vi "y轴排序.vi"(3 "均值角点":cluster{"X":sgl, "Y":sgl}[](array[cluster])) -> (1 "数组 2":cluster{"X":sgl, "Y":sgl}[](array[cluster]))   [LabVIEW 2018]
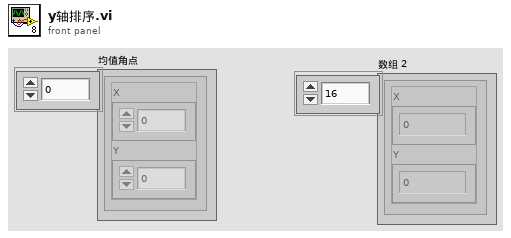
[diagram p1: front panel]
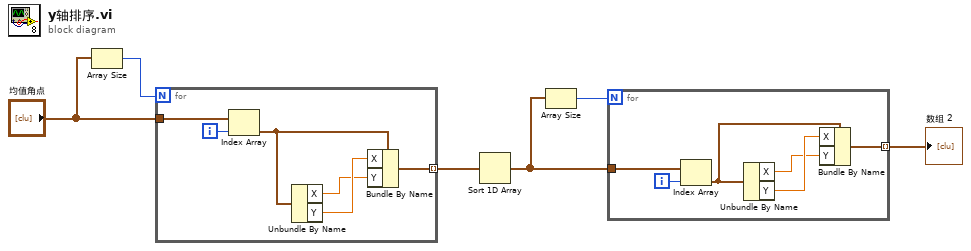
[diagram p0: block diagram]
diagram:
  n1 = Array Size(array="均值角点") -> (size(s)=w5:i32)
  n2 = for {
    N: w5 -> [_]
    tunnel: [w8] -> w4 mode=indexing
    tunnel: "均值角点" -> [w7]
    i -> [w12]
    n3 = Index Array(array=w7, index=w12) -> (element=w9:cluster{"X":sgl, "Y":sgl})
    n4 = Unbundle By Name(w9) -> ("X"=w10:sgl, "Y"=w11:sgl)
    n5 = Bundle By Name(cluster=w9, "X"=w11, "Y"=w10) -> (w8:cluster{"X":sgl, "Y":sgl})
  }
  n6 = Sort 1D Array(array=w4) -> (sorted array=w2:cluster{"X":sgl, "Y":sgl}[])
  n7 = Array Size(array=w2) -> (size(s)=w3:i32)
  n8 = for {
    N: w3 -> [_]
    tunnel: [w14] -> w1 mode=indexing
    tunnel: w2 -> [w13]
    i -> [w18]
    n9 = Index Array(array=w13, index=w18) -> (element=w15:cluster{"X":sgl, "Y":sgl})
    n10 = Unbundle By Name(w15) -> ("X"=w16:sgl, "Y"=w17:sgl)
    n11 = Bundle By Name(cluster=w15, "X"=w17, "Y"=w16) -> (w14:cluster{"X":sgl, "Y":sgl})
  }
  "数组 2" <- w1
